vi "FunctionSolverQuadraticDifferentiated.vi"(1 "x":dbl, 2 "b":dbl, 3 "a":dbl) -> (0 "f'(x)":dbl)   [LabVIEW 2021]
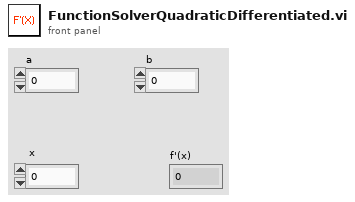
[diagram p1: front panel]
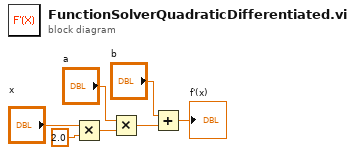
[diagram p0: block diagram]
diagram:
  n1 = Multiply(x="x", y=2.0) -> (x*y=w2:dbl)
  n2 = Multiply(x="a", y=w2) -> (x*y=w5:dbl)
  n3 = Add(x="b", y=w5) -> (x+y=→"f'(x)":dbl)
